vi "T from R.vi"(10 "R":sgl, 11 "Coefficients":dbl[](array[numeric])) -> (3 "T":sgl)   [LabVIEW 2014, in "Temperature.lvlib"]
uses:
  Temperature.lvlib
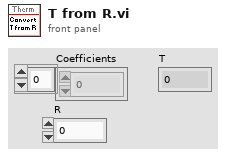
[diagram p1: front panel]
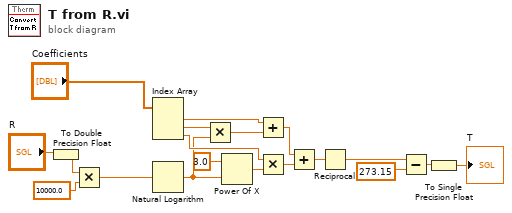
[diagram p0: block diagram]
diagram:
  n1 = To Double Precision Float(number="R") -> (double precision float=w17:dbl)
  n2 = Multiply(x=w17, y=10000.0) -> (x*y=w15:dbl)
  n3 = Index Array(array="Coefficients") -> (element #1=w2:dbl, element #2=w4:dbl, element #3=w7:dbl)  [unwired: 3 in]
  n4 = Natural Logarithm(1:w15) -> (0:w5:dbl)
  n5 = Multiply(x=w4, y=w5) -> (x*y=w6:dbl)
  n6 = Power Of X(1:w5, 2:3.0 ("y")) -> (0:w8:dbl)
  n7 = Add(x=w2, y=w6) -> (x+y=w10:dbl)
  n8 = Multiply(x=w7, y=w8) -> (x*y=w9:dbl)
  n9 = Add(x=w10, y=w9) -> (x+y=w11:dbl)
  n10 = Reciprocal(x=w11) -> (1/x=w12:dbl)
  n11 = Subtract(x=w12, y=273.15) -> (x-y=w18:dbl)
  n12 = To Single Precision Float(number=w18) -> (single precision float=→"T":sgl)
